vi "Set SpecimenTempCtrlParameter.vi"(7 "Specimen TempCtrl Parameter":T1, 8 "error in (no error)":errorcluster, 10 "Address (0)":i32, 11 "VISA resource name":refnum<visa-resource-name>) -> (0 "error out":errorcluster, 3 "VISA resource name out":refnum<visa-resource-name>)   [LabVIEW 2016, in "Environment Chamber.lvlib" / "Climatic Chamber.lvlib"]
doc: "<b>Specimen temperature control parameter setting</B>\n\nSets the specimen temperature control parameters.\n\n<b>Details:</b>s\n- Specify the upper limit from the chamber lower limit setting to the chamber upper limit setting.\n- Specify the lower limit from the chamber upper limit setting to the chamber lower limit setting.\n- Specify the P parameter from 0.0 to 100.0.\n- Specify the filter value from 0.0 to 1000.0.\n- Specify the I parameter from 0.0 to 1000.0.\n- Option setting 1 and option setting 2 are unused. Specify \"0\"."
uses:
  Climatic Chamber.lvlib
  Private/Type Defs/Specimen TempCtrl Settings Cluster.ctl
panel:
  out "NACK":bool
  out "Error":bool
  out "ACK":bool
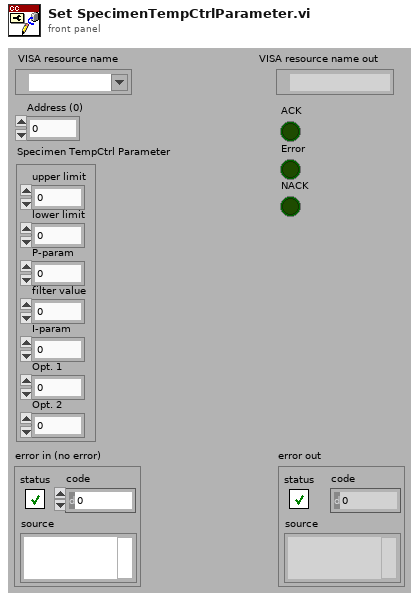
[diagram p1: front panel]
types:
  T1 = typedef "Environment Chamber.lvlib/Climatic Chamber.lvlib/Specimen TempCtrl Settings Cluster.ctl" = cluster{"upper limit":dbl, "lower limit":dbl, "P-param":dbl, "filter value":dbl, "I-param":dbl, "Opt. 1":dbl, "Opt. 2":dbl}
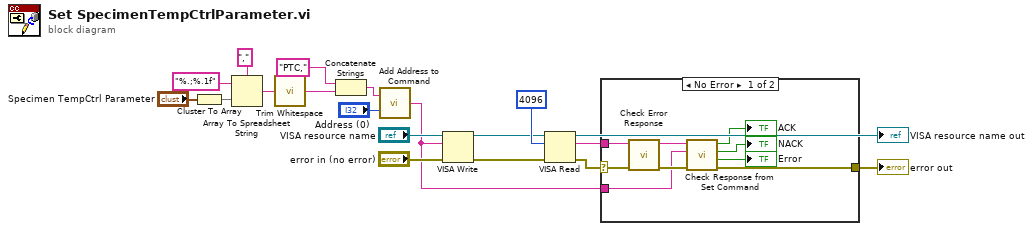
[diagram p0: block diagram]
diagram:
  n1 = Cluster To Array(cluster="Specimen TempCtrl Parameter") -> (array=w7:dbl[])
  n2 = Array To Spreadsheet String(delimiter (Tab)=",", array=w7, 3:"%.;%.1f" ("format string")) -> (spreadsheet string=w4:string)
  n3 = call <vilib>:"Trim Whitespace.vi"("string"=w4) -> ("trimmed string"=w3:string)  [unwired: 1 in]
  n4 = Concatenate Strings("PTC,", w3) -> (w1:string)
  n5 = call "Add Address to Command.vi"("Address (0)"="Address (0)", "Command"=w1) -> ("Command OUT"=w9:string)
  n6 = VISA Write(VISA resource name="VISA resource name", write buffer=w9, error in (no error)="error in (no error)") -> (VISA resource name out=w16:refnum<visa-resource-name>, error out=w15:errorcluster)  [unwired: 1 out]
  n7 = VISA Read(VISA resource name=w16, byte count=u32 4096, error in (no error)=w15) -> (VISA resource name out=→"VISA resource name out":refnum<visa-resource-name>, read buffer=w11:string, error out=w12:errorcluster)  [unwired: 1 out]
  n8 = case shown="No Error" w12 {
    selector: w12 -> [w27 w29]
    tunnel: w11 -> [w28 _]
    tunnel: [w23 w29] -> w10
    tunnel: w9 -> [w24 _]
    frame No Error {
      n9 = call "Check Error Response.vi"("error in (no error)"=w27, "read String"=w28) -> ("error out"=w26:errorcluster, "String out"=w25:string)  [unwired: 7 in, 1 out]
      n10 = call "Check Response from Set Command.vi"("error in (no error)"=w26, "Command"=w24, "Response"=w25) -> ("error out"=w23:errorcluster, "Error"=→"Error":bool, "NACK"=→"NACK":bool, "ACK"=→"ACK":bool)  [unwired: 5 in]
    }
    frame Error {
    }
  }
  "error out" <- w10
